vi "SaveFileType.vi"(0 "基路径":path, 1 "Save Type":string(combo)=".log", 2 "数值":i32, 3 "SN INPUT":string, 4 "PF":string) -> (14 "添加的路径":path, 15 "连接的字符串":string, 16 "数值 2":i32)   [LabVIEW 2018]
panel:
  out "字符串":string
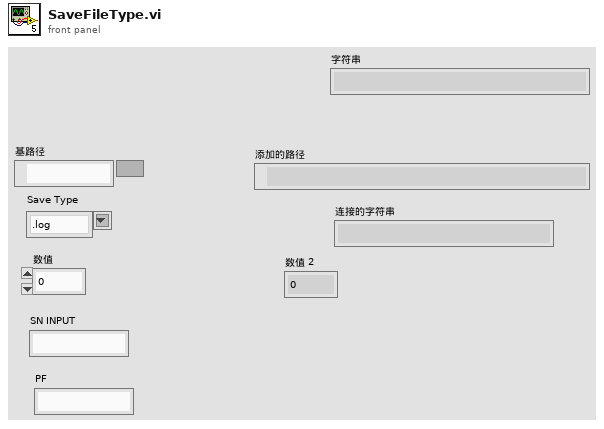
[diagram p1: front panel]
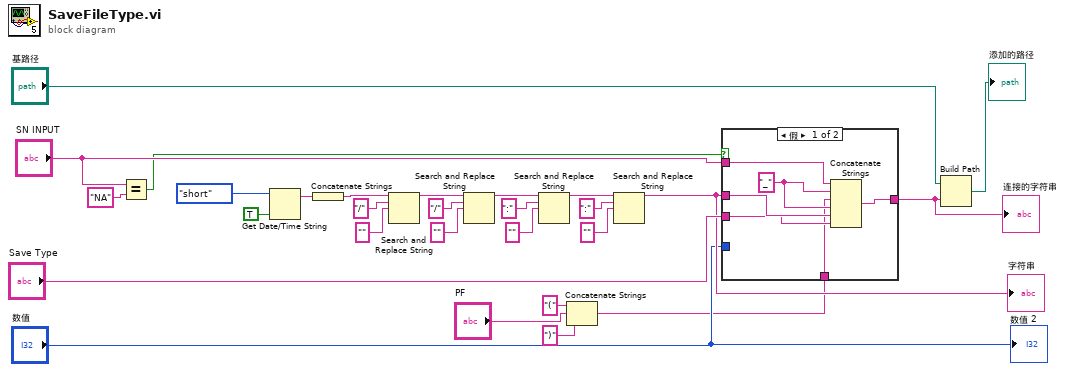
[diagram p0: block diagram]
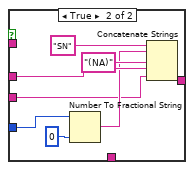
[diagram p2: hidden frame]
diagram:
  n1 = Equal?(x="SN INPUT", y="NA") -> (x = y?=w22:bool)
  n2 = Get Date/Time String(date format (0)=enum16{"short", "long", "abbreviated"}."short" ("日期格式(0)"), want seconds? (F)=TRUE ("需要秒？(F)")) -> (date string=w6:string)  [unwired: 1 in, 1 out]
  n3 = Concatenate Strings(w6) -> (w8:string)
  n4 = Search and Replace String(input string=w8, search string="/" ("搜索字符串"), replace string="" ("替换字符串(\"\")")) -> (result string=w13:string)  [unwired: 5 in, 3 out]
  n5 = Search and Replace String(input string=w13, search string="/" ("搜索字符串"), replace string="" ("替换字符串(\"\")")) -> (result string=w19:string)  [unwired: 5 in, 3 out]
  n6 = Search and Replace String(input string=w19, search string=":" ("搜索字符串"), replace string="" ("替换字符串(\"\")")) -> (result string=w14:string)  [unwired: 5 in, 3 out]
  n7 = Concatenate Strings("(" ("字符串"), "PF", ")" ("字符串")) -> (w1:string)
  n8 = Search and Replace String(input string=w14, search string=":" ("搜索字符串"), replace string="" ("替换字符串(\"\")")) -> (result string=w23:string)  [unwired: 5 in, 3 out]
  "字符串" <- w23
  n9 = case shown="假" w22 {
    tunnel: "数值" -> [_ w41]
    tunnel: w23 -> [w34 w40]
    tunnel: [w33 w39] -> w27
    tunnel: "SN INPUT" -> [w31 _]
    tunnel: "Save Type" -> [w32 w35]
    tunnel: w1 -> [w29 _]
    frame False {
      w30 = "_" ("字符串")
      n10 = Concatenate Strings(w31, w30, w29, w30, w34, w32) -> (w33:string)
    }
    frame True {
      n11 = Number To Fractional String(number=w41, precision (6)=i16 0 ("精度(6)")) -> (F-format string=w36:string)  [unwired: 2 in]
      n12 = Concatenate Strings("SN" ("字符串"), w36, "(NA)", w40, w35) -> (w39:string)
    }
  }
  "连接的字符串" <- w27
  n13 = Build Path(base path="基路径", name or relative path=w27) -> (appended path=→"添加的路径":path)
  "数值 2" <- "数值"
